vi "Indentify Hardware Type.vi"(8 "error in (no error)":errorcluster, 10 "Hw Info":T1) -> (0 "error out":errorcluster, 1 "String":string, 2 "Hardware Type":T2)   [LabVIEW 2020, in "Volatus.lvlib" / "Hardware Info Module.lvclass"]
uses:
  Hardware Info Module.lvclass
  Hardware Type.ctl
  HW Info.ctl
  Volatus.lvlib
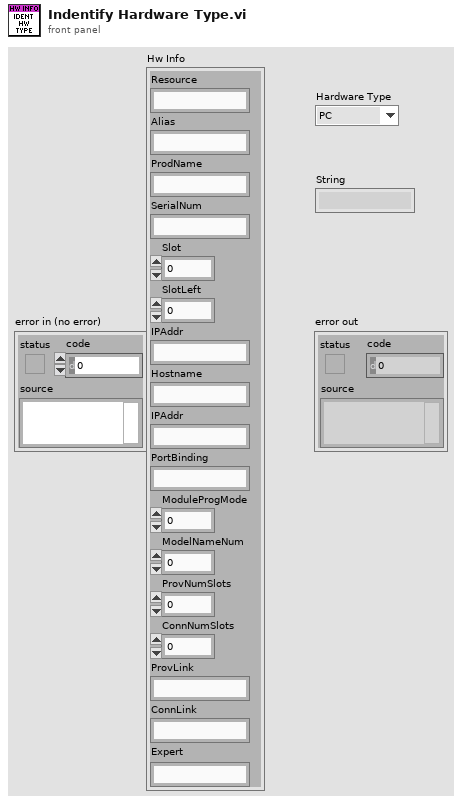
[diagram p1: front panel]
types:
  T1 = typedef "Volatus.lvlib/Hardware Info Module.lvclass/HW Info.ctl" = cluster{"Resource":string, "Alias":string, "ProdName":string, "SerialNum":string, "Slot":i32, "SlotLeft":u32, "IPAddr":string, "Hostname":string, "IPAddr":string, "PortBinding":string, "ModuleProgMode":u32, "ModelNameNum":u32, "ProvNumSlots":i32, "ConnNumSlots":i32, "ProvLink":string, "ConnLink":string, "Expert":string}
  T2 = typedef "Volatus.lvlib/Hardware Type.ctl" = enum16{"PC", "cRIO", "PXI"}
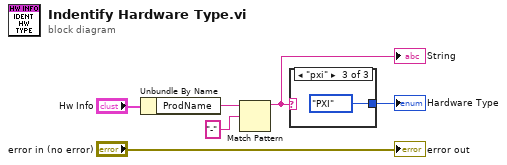
[diagram p0: block diagram]
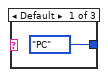
[diagram p2: hidden frame]
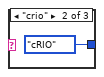
[diagram p3: hidden frame]
diagram:
  n1 = Unbundle By Name("Hw Info") -> ("ProdName"=w5:string)
  n2 = Match Pattern(string=w5, regular expression="-") -> (before substring=w3:string)  [unwired: 1 in, 3 out]
  "String" <- w3
  n3 = case shown="\"pxi\"" w3 {
    tunnel: [Hardware_Type."PC" ("Hardware Type") Hardware_Type."cRIO" ("Hardware Type") Hardware_Type."PXI" ("Hardware Type")] -> w2
    frame Default {
    }
    frame "crio" {
    }
    frame "pxi" {
    }
  }
  "Hardware Type" <- w2
  "error out" <- "error in (no error)"
